vi "lvssh2_session_callback_get_function.vi"(8 "error in (no error)":errorcluster, 11 "callback type":T1) -> (0 "error out":errorcluster, 3 "callback function":u64)   [LabVIEW 2017, in "libssh2.lvlib"]
uses:
  libssh2.lvlib
  libssh2_session_callback_type.ctl
  <vilib>/Utility/error.llb/Error Cluster From Error Code.vi
  <vilib>/ErrorRing/Error Ring.xnode
  lvssh2_extensions_64.dll
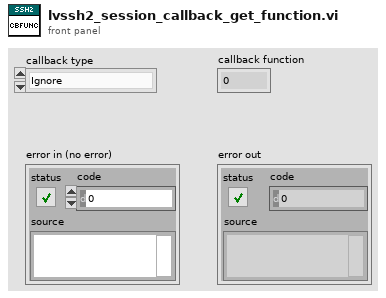
[diagram p1: front panel]
types:
  T1 = typedef "libssh2.lvlib/libssh2_session_callback_type.ctl" = enum16{"Ignore", "Debug", "Disconnect", "MAC Error", "X11", "Send", "Receive", "Auth Agent", "Auth Agent Identities", "Auth Agent Sign"}
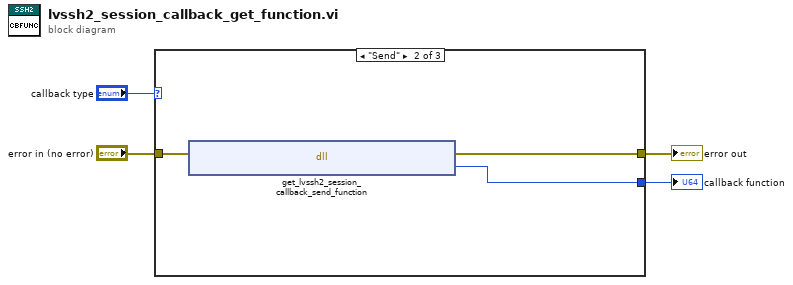
[diagram p0: block diagram]
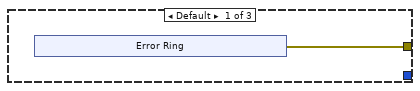
[diagram p2: hidden frame]
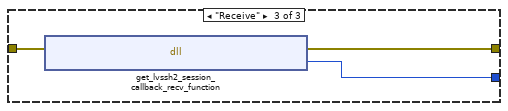
[diagram p3: hidden frame]
diagram:
  n1 = case shown="\"Send\"" "callback type" {
    tunnel: [_ w12 w15] -> w4
    tunnel: "error in (no error)" -> [_ w11 w14]
    tunnel: [w5 w10 w13] -> w1
    frame Default {
      n2 = xnode "Error Ring"() -> ("error out"=w5:errorcluster)
    }
    frame "Send" {
      n3 = dll-call lib="C:/Users/Pascal/Projects/Home/lvssh2/libssh2/lvssh2_extensions**.*" fn="get_lvssh2_session_callback_send_function"(error in=w11) -> (error out=w10:errorcluster, "return type"=w12:u64)  [unwired: 2 in, 1 out]
    }
    frame "Receive" {
      n4 = dll-call lib="C:/Users/Pascal/Projects/Home/lvssh2/libssh2/lvssh2_extensions**.*" fn="get_lvssh2_session_callback_recv_function"(error in=w14) -> (error out=w13:errorcluster, "return type"=w15:u64)  [unwired: 2 in, 1 out]
    }
  }
  "callback function" <- w4
  "error out" <- w1
